vi "VsEP-Plot Waveforms.vi"(0 "Array":dbl[][](array[numeric]), 1 "graph ref":refnum<vi>, 5 "dt (us)":dbl, 7 "Normalize traces":bool, 9 "Sequence values":dbl[](array[numeric]), 11 "error in (no error)":errorcluster, 12 "Max #SPL":i32, 13 "Position.X":dbl=-0.5) -> (4 "output cluster":cluster{i32, "dt (ms)":dbl, dbl[][]}, 15 "error out":errorcluster)   [LabVIEW 2020]
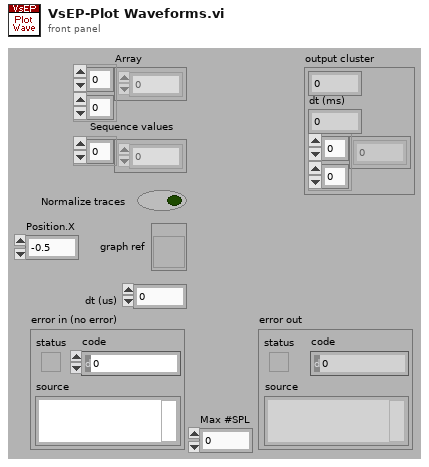
[diagram p1: front panel]
types:
  T1 = cluster{"Name":string, "Color":u32, "Style":u8, "Point Style":u8, "Name Visible":bool, "Allow Drag":bool, "Annotation Mode":u32, "Plot":i32, "Index":i32, "Position":cluster{"X":dbl, "Y":dbl}, "X Scale":u32, "Y Scale":u32, "Show Arrow":bool, "Lock Name":bool, "Plot Area":i32, "Label Offset":cluster{"X":dbl, "Y":dbl}}
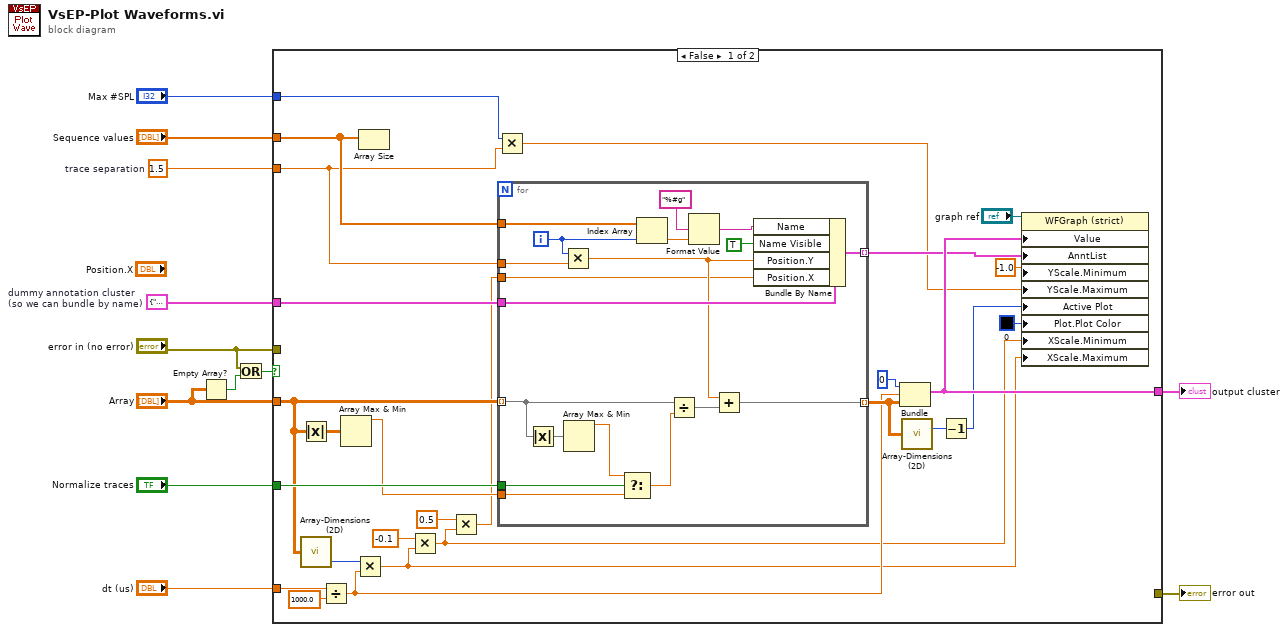
[diagram p0: block diagram]
diagram:
  w7 = 1.5  # trace separation
  w9 = T1 {"Name"="", "Color"=0, "Style"=0, "Point Style"=0, "Name Visible"=FALSE, "Allow Drag"=FALSE, "Annotation Mode"=0, "Plot"=0, "Index"=0, "Position"={"X"=0.0, "Y"=0.0}, "X Scale"=0, "Y Scale"=0, "Show Arrow"=FALSE, "Lock Name"=FALSE, "Plot Area"=0, "Label Offset"={"X"=0.0, "Y"=0.0}}  # dummy annotation cluster (so we can bundle by name)
  n1 = Empty Array?(array="Array") -> (empty?=w4:bool)
  n2 = Or(x="error in (no error)", y=w4) -> (x .or. y?=w2:bool)
  n3 = case shown="False" w2 {
    tunnel: [w35 _] -> w12
    tunnel: "Array" -> [w20 _]
    tunnel: "dt (us)" -> [w38 _]
    tunnel: [_ w59] -> w10
    tunnel: "Sequence values" -> [w31 _]
    tunnel: w9 -> [w34 _]
    tunnel: w7 -> [w30 _]
    tunnel: "Normalize traces" -> [w28 _]
    tunnel: "Max #SPL" -> [w25 _]
    tunnel: "error in (no error)" -> [_ w59]
    frame False {
      n4 = Absolute Value(x=w20) -> (abs(x)=w27:dbl[][])
      n5 = call "Array-Dimensions (2D).vi"("2D Array"=w20) -> ("# columns"=w19:i32)  [unwired: 13 in, 1 out]
      n6 = Divide(x=w38, y=1000.0) -> (x/y=w18:dbl)
      n7 = Array Max & Min(array=w27) -> (max value=w26:dbl)  [unwired: 3 out]
      n8 = Multiply(x=w19, y=w18) -> (x*y=w17:dbl)
      n9 = Array Size(array=w31) -> ()  [unwired: 1 out]
      n10 = Multiply(x=-0.1, y=w17) -> (x*y=w13:dbl)
      n11 = Multiply(x=0.5, y=w13) -> (x*y=w14:dbl)
      n12 = Multiply(x=w25, y=w30) -> (x*y=w29:dbl)
      n13 = for {
        tunnel: w20 -> [w56] mode=indexing
        tunnel: [w57] -> w24 mode=indexing
        tunnel: w31 -> [w54]
        tunnel: w34 -> [w53]
        tunnel: [w48] -> w33 mode=indexing
        tunnel: w30 -> [w47]
        tunnel: w28 -> [w44]
        tunnel: w26 -> [w41]
        tunnel: w14 -> [w40]
        i -> [w52]
        n14 = Absolute Value(x=w56) -> (abs(x)=w58:dbl[])
        n15 = Multiply(x=w52, y=w47) -> (x*y=w46:dbl)
        n16 = Array Max & Min(array=w58) -> (max value=w43:dbl)  [unwired: 3 out]
        n17 = Select(t=w43, s=w44, f=w41) -> (s? t:f=w42:dbl)
        n18 = Index Array(array=w54, index=w52) -> (element=w51:dbl)
        n19 = Divide(x=w56, y=w42) -> (x/y=w45:dbl[])
        n20 = Format Value(format string="%#g", value (0)=w51) -> (output string=w49:string)  [unwired: 1 in]
        n21 = Add(x=w46, y=w45) -> (x+y=w57:dbl[])
        n22 = Bundle By Name(cluster=w53, "Name"=w49, "Name Visible"=TRUE, "Position.Y"=w46, "Position.X"=w40) -> (w48:T1)
      }
      n23 = Bundle(0, w18, w24) -> (w35:cluster{i32, dbl, dbl[][]})  [unwired: 1 in]
      n24 = call "Array-Dimensions (2D).vi"("2D Array"=w24) -> ("# rows"=w23:i32)  [unwired: 13 in, 1 out]
      n25 = Decrement(x=w23) -> (x-1=w22:i32)
      n26 = property class="WFGraph (strict)"(reference="graph ref", "Value"=w35, "AnntList"=w33, "YScale.Minimum"=-1.0 ("Y Scale.Range:Minimum"), "YScale.Maximum"=w29, "Active Plot"=w22, "Plot.Plot Color"=u32 0, "XScale.Minimum"=w13, "XScale.Maximum"=w17) -> ()  [unwired: 1 in, 2 out]
    }
    frame True {
    }
  }
  "output cluster" <- w12
  "error out" <- w10
